vi "Write FP Control.vi"(8 "error in (no error)":errorcluster, 9 "Control Value":variant, 10 "Control Name":string="Parameters", 11 "Mag Lab Measure Base in":refnum<class "Mag Lab Measure Base.lvclass">) -> (0 "error out":errorcluster, 3 "Mag Lab Measure Base out":refnum<class "Mag Lab Measure Base.lvclass">)   [LabVIEW 2015, in "Mag Lab Measure Base.lvclass"]
uses:
  Mag Lab Measure Base.lvclass
  Mag Lab Root/Mag Lab Root.lvclass/Mag Lab Root.ctl
  Mag Lab Root/Read Front Panel ref.vi
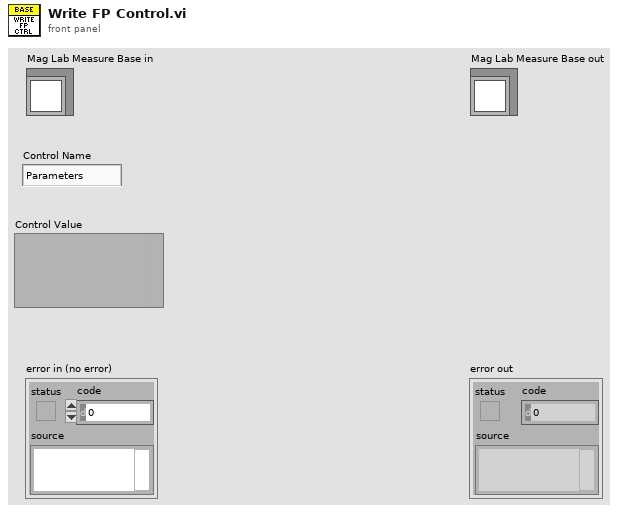
[diagram p1: front panel]
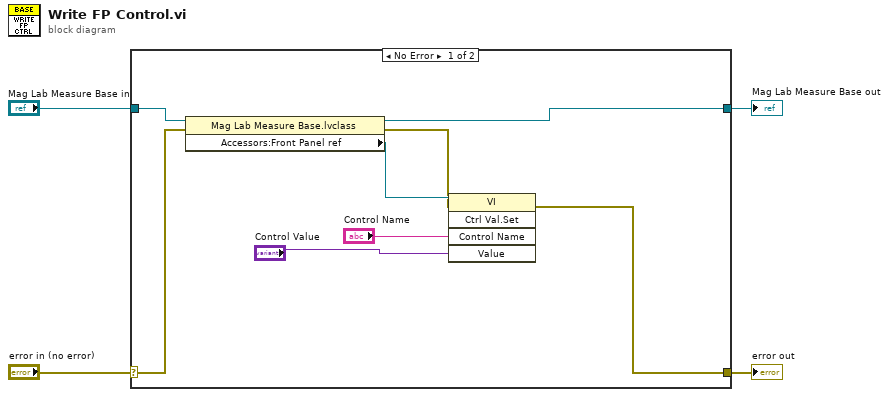
[diagram p0: block diagram]
diagram:
  n1 = case shown="No Error" "error in (no error)" {
    selector: "error in (no error)" -> [w6 w14]
    tunnel: [w9 w14] -> w3
    tunnel: [w8 w13] -> w1
    tunnel: "Mag Lab Measure Base in" -> [w12 w13]
    frame No Error {
      n2 = property class="Mag Lab Measure Base.lvclass"(reference=w12, error in=w6) -> (reference out=w8:refnum<class "Mag Lab Measure Base.lvclass">, error out=w5:errorcluster, "Accessors:Front Panel ref"=w7:refnum<vi>)
      n3 = invoke class="VI" method="Ctrl Val.Set"(reference=w7, error in=w5, "Control Name"="Control Name", "Value"="Control Value") -> (error out=w9:errorcluster)  [unwired: 1 in, 4 out]
    }
    frame Error {
    }
  }
  "error out" <- w3
  "Mag Lab Measure Base out" <- w1
